vi "Obtain Actual Voltage.vi"(8 "Error In":errorcluster, 10 "Error Percentage":dbl format="%#_13g", 11 "ADC in":refnum<class "ADC.lvclass">) -> (0 "Error Out":errorcluster, 3 "ADC out":refnum<class "ADC.lvclass">)   [LabVIEW 2023, in "ADC.lvclass"]
uses:
  ADC.lvclass
  C:/Users/ancya/Downloads/Assignment 4/Assignment 4/SDLC - DNL and INL Testing/INL DNL/Classes/Mode/Mode.lvclass
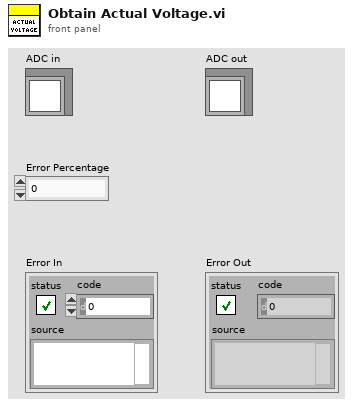
[diagram p1: front panel]
types:
  T1 = typedef "Transfer Function.ctl" = cluster{"Ideal voltage":dbl[], "Digital Code":dbl[]}
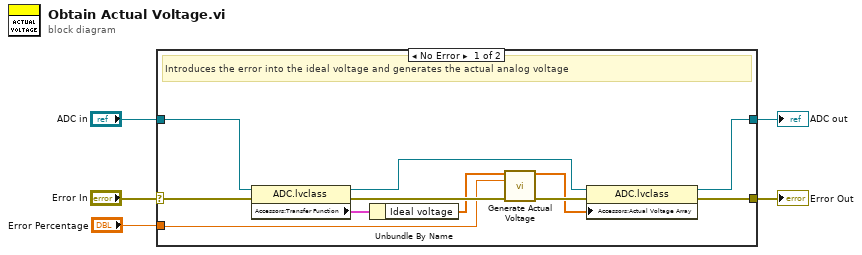
[diagram p0: block diagram]
diagram:
  n1 = case shown="No Error" "Error In" {
    selector: "Error In" -> [w16 w18]
    tunnel: [w9 w18] -> w4
    tunnel: [w6 w17] -> w2
    tunnel: "ADC in" -> [w13 w17]
    tunnel: "Error Percentage" -> [w10 _]
    frame No Error {
      # "Introduces the error into the ideal voltage and generates the actual analog voltage"
      n2 = property class="ADC.lvclass"(reference=w13, error in=w16) -> (reference out=w8:refnum<class "ADC.lvclass">, error out=w14:errorcluster, "Accessors:Transfer Function"=w12:T1)
      n3 = Unbundle By Name(w12) -> ("Ideal voltage"=w11:dbl[])
      n4 = call "Generate Actual Voltage.vi"("VoltageArray"=w11, "ErrorValue"=w10, "error in"=w14) -> ("ActualVoltageArray"=w7:dbl[], "error out"=w15:errorcluster)  [unwired: 11 in]
      n5 = property class="ADC.lvclass"(reference=w8, error in=w15, "Accessors:Actual Voltage Array"=w7) -> (reference out=w6:refnum<class "ADC.lvclass">, error out=w9:errorcluster)
    }
    frame Error {
    }
  }
  "Error Out" <- w4
  "ADC out" <- w2
